vi "TMN_Query.vi"(0 "System no.":i32=1 min=1 max=4 step=1, 2 "Axes to query":string[](array[string]), 3 "All axes?":bool, 4 "Axis identifier?":bool=TRUE, 5 "error in":errorcluster) -> (14 "Minimum travel limit":dbl[](array[numeric]) format="%.6f", 19 "error out":errorcluster)   [LabVIEW 2020]
doc: "Returns minimum (low-end) travel limit (if present, position of negative limit switch, or value of negative soft limit, if set, whichever is higher).\n\nAnalog, C-413, C-702, C-848, C-865, C-866, C-867, C-877, C-880, C-884, C-885, C-887, C-891, E-517, E-518, E-709, E-712, E-725, E-727, E-753, E-754, E-761, E-861, E-871, E-873, E-874, F-206, Hydra, Pollux, M-8X0, Mercury, Mercury_GCS: If All axes? = TRUE, then Axis identifier? can be FALSE\n\nC-843, C-843.PM, C-844, E-710: If All axes? = TRUE, then Axis identifier? must be TRUE\n\nC-413, C-867, C-877, C-884, C-891, E-861, E-871, E-873, E-874, Hydra, Pollux, Mercury_GCS: If All axes? = TRUE, then Axis identifier? can be FALSE. The minimum commandable position is defined by the MAX_TRAVEL_RANGE_NEG parameter ID 0x30 (SPA).\n\nE-755: If All axes? = TRUE, then Axis identifier? can be FALSE. Command not available for E-755.101.\n\nE-517, E-761: If All axes? = TRUE, then Axis identifier? can be FALSE. Get the maximum accessible position value, i.e. the value of the \"Range max limit\" parameter (ID 0x07000001). Note: The maximum position which can be commanded depends either on the \"Range max limit\" parameter or-if it is smaller than the \"Range max limit\" parameter value- on the value of the positive soft limit set with PLM.\n\nC-887, F-206, M-8X0: Only for GCS syntax version = GCS 2.0 or higher (Check with CSV?.vi. If CSV?.vi is not supported, syntax version is GCS 1.0). TMN? returns the minimum travel range of the axis with all other axes positions being zero. If this is not the case, the available travel range may be less."
panel:
  # "Returns minimum travel limit (position of negative limit switch,\nor value of negative soft limit, if set, whichever is higher)."
  # "If all axes: use"
  # "Query"
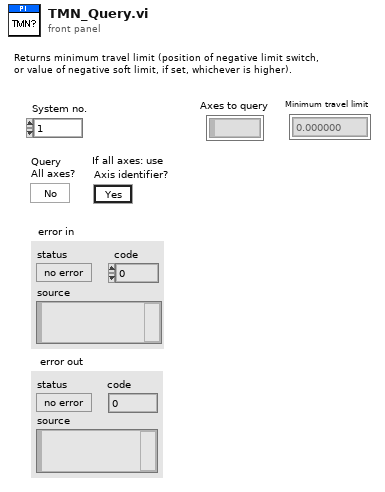
[diagram p1: front panel]
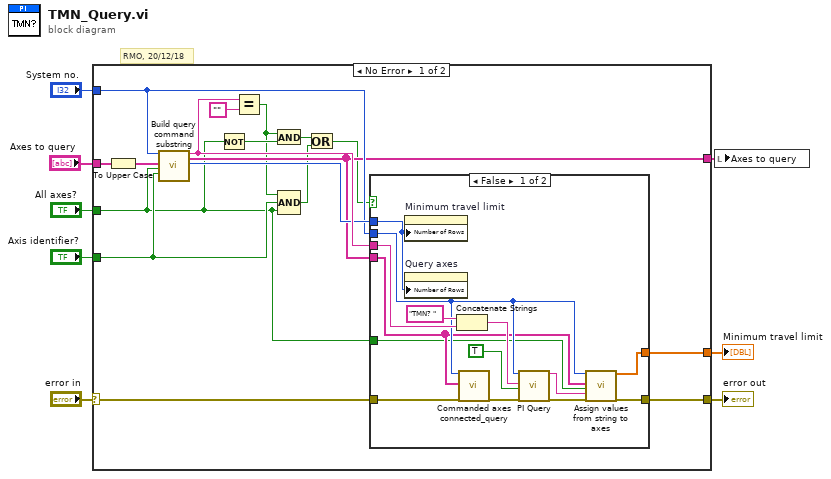
[diagram p0: block diagram]
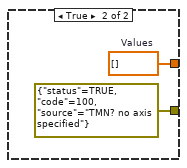
[diagram p2: hidden frame]
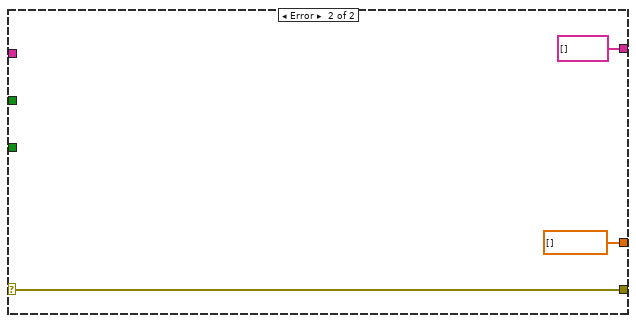
[diagram p3: hidden frame]
diagram:
  # "RMO, 20/12/18"
  n1 = case shown="No Error" "error in" {
    selector: "error in" -> [w11 w42]
    tunnel: [w25 dbl[] [] ("Values")] -> w8
    tunnel: "Axes to query" -> [w24 _]
    tunnel: [w10 w42] -> w6
    tunnel: "System no." -> [w19 _]
    tunnel: [w18 string[] [] ("Axes to query out")] -> w4
    tunnel: "Axis identifier?" -> [w14 _]
    tunnel: "All axes?" -> [w13 _]
    frame No Error {
      n2 = To Upper Case(1:w24) -> (0:w22:string[])
      n3 = call "Build query command substring.vi"("System no."=w19, "Axes to query in"=w22, "Query\nAll axes?"=w13, "For all axes: use\nAxis identifier?"=w14) -> ("Command substring"=w21:string, "Axes to query out"=w18:string[], "Number of rows"=w20:u32)  [unwired: 2 in, 11 out]
      n4 = Not(x=w13) -> (.not. x?=w17:bool)
      n5 = Equal?(x=w21, y="" ("x")) -> (x = y?=w15:bool)
      n6 = And(x=w15, y=w17) -> (x .and. y?=w16:bool)
      n7 = Compound Arithmetic op=AND(w15, w14, w13) -> (w12:bool)
      n8 = Or(x=w16, y=w12) -> (x .or. y?=w9:bool)
      n9 = case shown="False" w9 {
        tunnel: [w36 w40] -> w25
        tunnel: w21 -> [w35 _]
        tunnel: w20 -> [w34 _]
        tunnel: w19 -> [w33 _]
        tunnel: w18 -> [w32 _]
        tunnel: w13 -> [w31 _]
        tunnel: w11 -> [w29 _]
        tunnel: [w28 errorcluster {"status"=TRUE, "code"=100, "source"="TMN? no axis specified"} ("error out")] -> w10
        frame False {
          n10 = property on="Minimum travel limit" class="Arr (strict)"("Number of Rows"=w34) -> ()  [unwired: 2 in, 2 out]
          n11 = property on="Query axes" class="Arr (strict)"("Number of Rows"=w34) -> ()  [unwired: 2 in, 2 out]
          n12 = Concatenate Strings("TMN? ", w35) -> (w37:string)
          n13 = call "Commanded axes connected_query.vi"("System no."=w33, "Commanded axes"=w32, "error in"=w29) -> ("error out"=w30:errorcluster)  [unwired: 1 in, 15 out]
          n14 = call "PI Query.vi"("System no."=w33, "String to send"=w37, "Attach termination char.?"=TRUE ("Attach Linefeed?"), "error in"=w30) -> ("String read"=w26:string, "error out"=w27:errorcluster)  [unwired: 3 in, 11 out]
          n15 = call "Assign values from string to axes.vi"("System no."=w33, "Queried axes"=w32, "All axes queried?"=w31, "Input String"=w26, "error in"=w27) -> ("Values"=w36:dbl[], "error out"=w28:errorcluster)  [unwired: 4 in, 9 out]
        }
        frame True {
          w40 = dbl[] []  # Values
        }
      }
    }
    frame Error {
    }
  }
  "error out" <- w6
  "Minimum travel limit" <- w8
  n16 = local write "Axes to query"(w4) -> ()
